vi "Create RF Waveform Database.vi"(8 "error in (no error)":errorcluster, 11 "QPA Measurement in":refnum<class "QPA Measurement.lvclass">) -> (0 "error out":errorcluster, 3 "QPA Measurement out":refnum<class "QPA Measurement.lvclass">)   [LabVIEW 2016, in "QPA Measurement.lvlib" / "QPA Measurement.lvclass"]
uses:
  QPA Measurement.lvclass
  C:/Projects/STS/Common/Sequence Automation/Plugins/Measurement Interface.lvlibp/Measurement Interface.lvclass
  QPA Measurement.lvclass/QPA Measurement.ctl
  Plugins/Measurement Interface.lvlibp/Private Methods/Active Sequence File/Read Active Sequence File.vi
  Waveform Manager/QPA MSMT Waveform Manager.lvclass
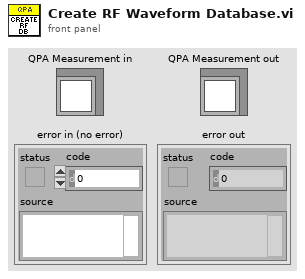
[diagram p1: front panel]
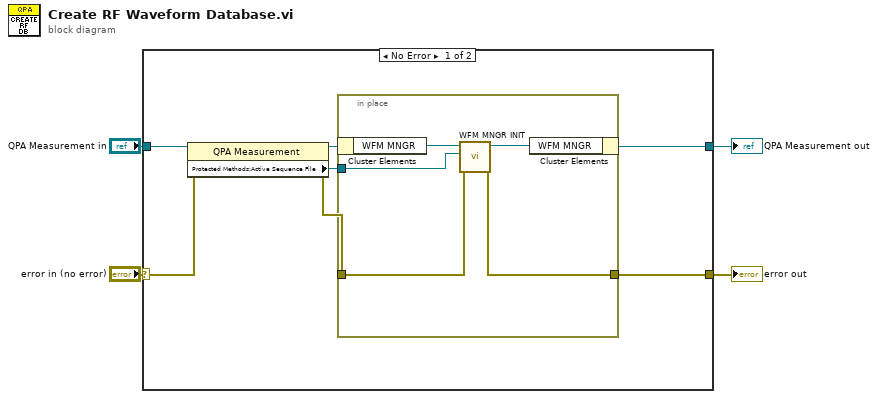
[diagram p0: block diagram]
diagram:
  n1 = case shown="No Error" "error in (no error)" {
    selector: "error in (no error)" -> [w11 w18]
    tunnel: [w7 w18] -> w3
    tunnel: [w5 w17] -> w1
    tunnel: "QPA Measurement in" -> [w10 w17]
    frame No Error {
      n2 = property class="QPA Measurement"(reference=w10, error in=w11) -> (reference out=w6:refnum<class "QPA Measurement.lvclass">, error out=w8:errorcluster, "Protected Methods:Active Sequence File"=w9:refnum<k7>)
      n3 = in-place {
        in-place-border: w9 -> [w14]
        in-place-border: w8 -> [w13]
        in-place-border: [w12] -> w7
        n4 = in-place-cluster #1(w6) -> ("WFM MNGR"=w16:refnum<class "QPA MSMT Waveform Manager.lvclass">)
        n5 = call "WFM MNGR INIT.vi"("error in (no error)"=w13, "Sequence File"=w14, "WFM MNGR in"=w16) -> ("error out"=w12:errorcluster, "WFM MNGR out"=w15:refnum<class "QPA MSMT Waveform Manager.lvclass">)  [unwired: 7 in]
        n6 = in-place-cluster #1("WFM MNGR"=w15) -> (w5:refnum<class "QPA Measurement.lvclass">)
      }
    }
    frame Error {
    }
  }
  "error out" <- w3
  "QPA Measurement out" <- w1
